vi "Write UI Objects.vi"(8 "error in (no error)":errorcluster, 10 "UI Objects":refnum<class "UI Object.lvclass">[](array[class]), 11 "Draw in":refnum<class "Draw.lvclass">) -> (0 "error out":errorcluster, 3 "Draw out":refnum<class "Draw.lvclass">)   [LabVIEW 2016, in "PacManClasses.lvlib" / "Draw.lvclass"]
uses:
  Draw.lvclass
  Geometric Figure/UI Object.lvclass
  Draw.lvclass/Draw.ctl
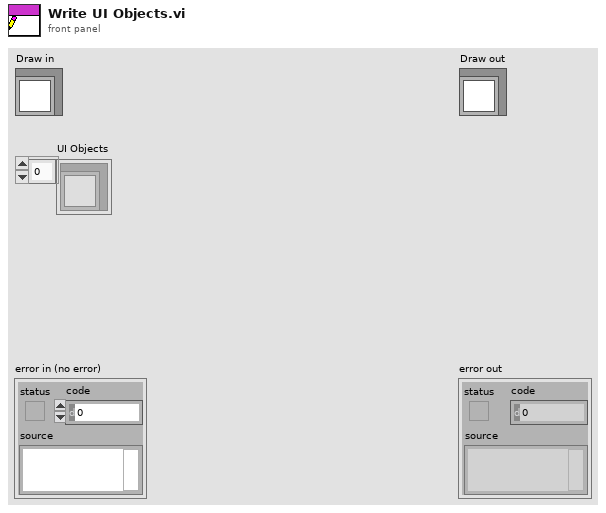
[diagram p1: front panel]
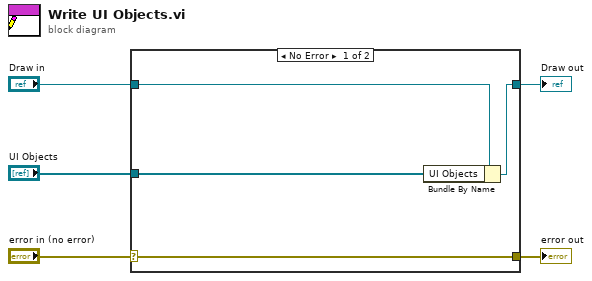
[diagram p0: block diagram]
diagram:
  n1 = case shown="No Error" "error in (no error)" {
    selector: "error in (no error)" -> [w9 w10]
    tunnel: [w9 w10] -> w4
    tunnel: [w7 w11] -> w2
    tunnel: "Draw in" -> [w8 w11]
    tunnel: "UI Objects" -> [w6 _]
    frame No Error {
      n2 = Bundle By Name(cluster=w8, "UI Objects"=w6) -> (w7:refnum<class "Draw.lvclass">)
    }
    frame Error {
    }
  }
  "error out" <- w4
  "Draw out" <- w2
